vi "PLC.CheckLiveBit.vi"(0 "LifeBit":bool, 1 "Timer [s] (3)":dbl=3.0) -> (2 "LiveBitElapsed":bool)   [LabVIEW 2016]
panel:
  out "LiveBitDuration":dbl
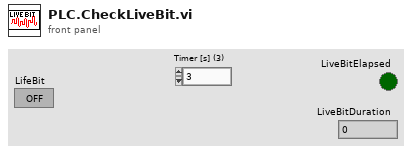
[diagram p1: front panel]
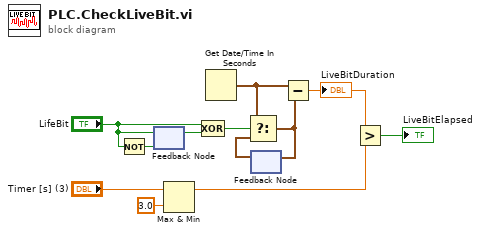
[diagram p0: block diagram]
diagram:
  n1 = Not(x="LifeBit") -> (.not. x?=w5:bool)
  n2 = feedback-in #1("LifeBit") -> ()
  n3 = feedback #1(w5) -> (w12:bool)
  n4 = Max & Min(x="Timer [s] (3)", y=3.0) -> (max(x,y)=w2:dbl)  [unwired: 1 out]
  n5 = Compound Arithmetic op=XOR("LifeBit", w12) -> (w11:bool)
  n6 = Get Date/Time In Seconds() -> (seconds since 1Jan1904=w8:timestamp)
  n7 = feedback #2() -> (w10:timestamp)  [unwired: 1 in]
  n8 = Select(t=w8, s=w11, f=w10) -> (s? t:f=w9:timestamp)
  n9 = feedback-in #2(w9) -> ()
  n10 = Subtract(x=w8, y=w9) -> (x-y=w7:dbl)
  "LiveBitDuration" <- w7
  n11 = Greater?(x=w7, y=w2) -> (0:→"LiveBitElapsed":bool)
